vi "IndicatorVI.vi"(3 "ChannelStatus":string) -> (0 "Array":bool[](array[boolean]))   [LabVIEW 2019]
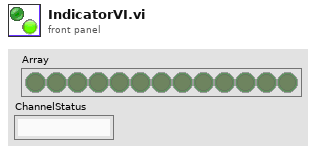
[diagram p1: front panel]
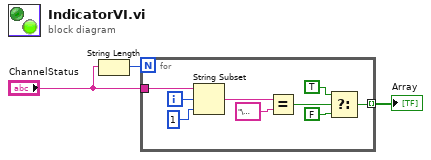
[diagram p0: block diagram]
diagram:
  n1 = String Length(string="ChannelStatus") -> (length=w3:i32)
  n2 = for {
    N: w3 -> [_]
    tunnel: "ChannelStatus" -> [w12]
    tunnel: [w5] -> w2 mode=indexing
    i -> [w4]
    n3 = String Subset(string=w12, offset (0)=w4, length (rest)=1 ("length (rest)")) -> (substring=w10:string)
    n4 = Equal?(x=w10, y="\u0001") -> (x = y?=w8:bool)
    n5 = Select(t=TRUE, s=w8, f=FALSE) -> (s? t:f=w5:bool)
  }
  "Array" <- w2
